vi "Subvi flush pixel clock.vi"   [LabVIEW 2017]
uses:
  Detector/GV N pixel clock per line.vi
  <vilib>/rvi/Memory/Memory_Emulation/nirvimemoryFastEmulation.vi
  <vilib>/rvi/Memory/Memory_Emulation/nirvimemoryEmulation.vi
  <vilib>/rvi/Emulation/niFpgaEmulationIsFPGAContextNoSignature.vi
  <vilib>/rvi/DataTransferAndStorage/Container/Common/niFpgaContainerGetUniqueNameForEmu.vi
  <vilib>/rvi/Emulation/niFpgaProcessEmulError.vi
  <vilib>/rvi/Emulation/niFpgaSctlEmulationGetInTimedLoop.vi
  <vilib>/rvi/errors/nirviReportUnexpectedCaseInternalError (U32).vi
  <vilib>/rvi/DataTransferAndStorage/Container/XNode/niFpgaContainer.xnode
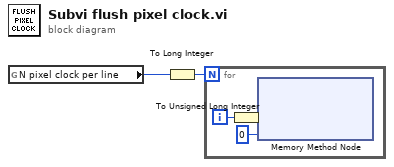
[diagram p0: block diagram]
diagram:
  n1 = global read "GV N pixel clock per line.vi" "N pixel clock per line"() -> (w1:i16)
  n2 = To Long Integer(number=w1) -> (32bit integer=w2:i32)
  n3 = for {
    N: w2 -> [_]
    i -> [w5]
    n4 = To Unsigned Long Integer(number=w5) -> (unsigned 32bit integer=w3:u32)
    n5 = xnode ("Memory Method Node")("Address"=w3, "Data"=u32 0) -> ()  [unwired: 1 in, 1 out]
  }
